vi "dll.set.vi"(8 "error in (no error)":errorcluster, 10 "dll":path, 11 "LabVIEW-MIDI-XPLAT in":refnum<class "LabVIEW-MIDI-XPLAT.lvclass">) -> (0 "error out":errorcluster, 3 "LabVIEW-MIDI-XPLAT out":refnum<class "LabVIEW-MIDI-XPLAT.lvclass">)   [LabVIEW 2020, in "LabVIEW-MIDI-XPLAT.lvclass"]
uses:
  LabVIEW-MIDI-XPLAT.lvclass
  LabVIEW-MIDI-XPLAT.lvclass/LabVIEW-MIDI-XPLAT.ctl
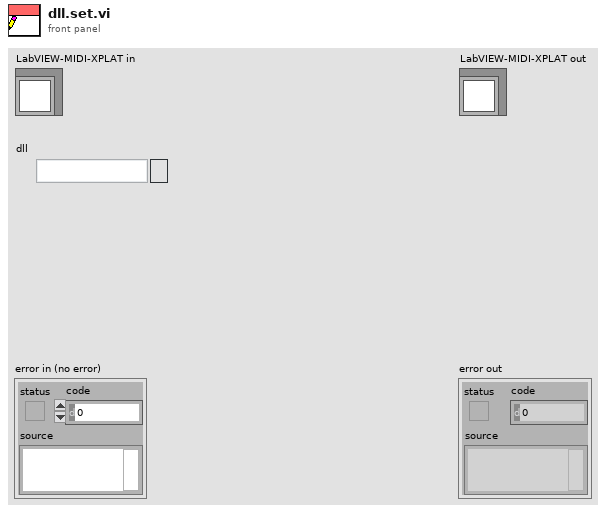
[diagram p1: front panel]
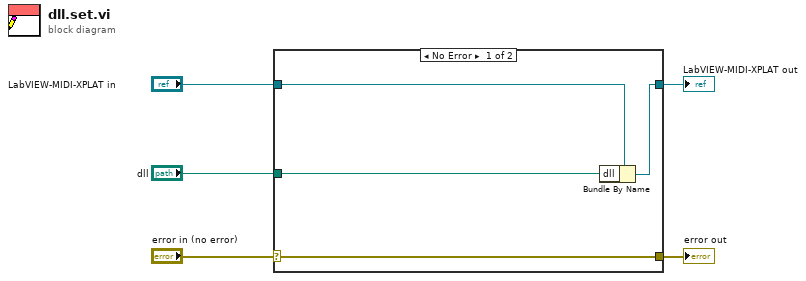
[diagram p0: block diagram]
diagram:
  n1 = case shown="No Error" "error in (no error)" {
    selector: "error in (no error)" -> [w9 w10]
    tunnel: [w9 w10] -> w4
    tunnel: [w7 w11] -> w2
    tunnel: "LabVIEW-MIDI-XPLAT in" -> [w8 w11]
    tunnel: "dll" -> [w6 _]
    frame No Error {
      n2 = Bundle By Name(cluster=w8, "dll"=w6) -> (w7:refnum<class "LabVIEW-MIDI-XPLAT.lvclass">)
    }
    frame Error {
    }
  }
  "error out" <- w4
  "LabVIEW-MIDI-XPLAT out" <- w2
